vi "SMR_LabVIEW_V8.4.vi"() -> ()   [LabVIEW 2025]
uses:
  <vilib>/DAQmx/write.llb/DAQmx Write (Analog DBL 1Chan 1Samp).vi
  <vilib>/DAQmx/read.llb/DAQmx Read (Analog 1D DBL NChan 1Samp).vi
  <vilib>/DAQmx/read.llb/DAQmx Read (Analog 2D DBL NChan NSamp).vi
  <vilib>/Analysis/baseanly.llb/Mean (DBL).vi
  <vilib>/DAQmx/create/channels.llb/DAQmx Create Channel (AI-Temperature-Thermocouple).vi
  <vilib>/DAQmx/create/channels.llb/DAQmx Create Channel (AI-Voltage-Basic).vi
  <vilib>/DAQmx/create/channels.llb/DAQmx Create Channel (AO-Voltage-Basic).vi
  <vilib>/DAQmx/miscellaneous.llb/DAQmx Fill In Error Info.vi
  <vilib>/DAQmx/configure/timing.llb/DAQmx Timing (Sample Clock).vi
  <vilib>/addons/control/pid/pid.llb/PID (DBL).vi
  <vilib>/measure/maspectr.llb/FFT Power Spectrum and PSD for 1 Chan.vi
  <vilib>/measure/matone.llb/Extract Single Tone Information 1 Chan.vi
  <vilib>/addons/control/pid/NI_PID_pid.lvlib
  <vilib>/Analysis/NI_AALBase.lvlib
  <vilib>/ptbypt/NI_PtbyPt.lvlib
  <vilib>/measure/NI_MAPro.lvlib
panel:
  out "HW Valve Command (V)":dbl
  in  "HX Flow Setpoint (GPM)":dbl
  in  "Manual HW Valve Voltage (V)":dbl
  in  "HW Valve: Manual / PID":bool
  in  "PID gains for HW Valve":T1={"proportional gain (Kc)"=1.0, "integral time (Ti, min)"=0.01, "derivative time (Td, min)"=0.0} {"derivative time (Td, min)" format="%.3f"; "integral time (Ti, min)" format="%.3f"; "proportional gain (Kc)" format="%.3f"}
  out "Rod Power (W)":dbl
  out "Current Through Rod (A)":dbl
  out "Time in Steady State (s)":dbl
  in  "Steady-State Dwell (s)":dbl
  out "Main Loop Flow (GPM)":dbl
  out "FM Amplitude":dbl
  out "FM Frequency":dbl
  out "Spectrum":cluster{"f0":dbl, "df":dbl, "magnitude":dbl[]}(graph)
  out "Raw Signal":waveform(dbl)(graph)
  out "Smoothed HX Flow (GPM)":dbl
  out "Flow History":dbl(graph)
  out "HX Flow (GPM)":dbl
  out "Voltage Across Rod (V)":dbl format="%0.2f"
  out "Current Run Folder":path
  in  "Log Root Folder":path=path "C:/Users/LocalUser/Documents/GitHub/thermal-loop/resources/v0.1.1/data/001"
  out "Raw NI9201 \nVoltage Display":T2
  in  "Loop Period (ms)":dbl=1000.0
  in  "Stop":bool
  out "Auto Steady State Threshold (deg C/min)":dbl
  out "Max dT/dt (deg C/min)":dbl
  out "Temp Change Rate (deg C/min)":dbl
  out "5-Min Baseline Complete":bool
  out "Rate Window Ready":bool
  out "Steady State":bool
  in  "Voltage Limit (V)":dbl=10.0
  in  "Temperature Limit (C)":dbl=50.0
  in  "Pressure Limit (psi)":dbl=15.0
  out "Max Voltage":bool
  out "Max Temperature":bool
  out "Max Pressure":bool
  out "Heat Exchanger Pressure History":dbl(graph)
  out "Main Loop Pressure History":T3(graph)
  out "Overall Avg Pressure (psi)":dbl
  out "Heat Exchanger Pressure P6 (psi)":dbl
  out "Main Loop Avg Pressure (psi)":dbl
  out "Pressure Display":T4
  out "Overall Pressure History":T5(graph)
  out "Max Loop Pressure (psi)":dbl
  out "Heat Exchanger Temperature History":cluster{"Waveform":dbl, "Waveform":dbl}(graph)
  out "Main Loop Temeperature History":T6(graph)
  out "Heat Exchanger Avg Temp (deg C)":dbl
  out "Temperature Display":T7
  out "Overall Temperature History":T8(graph)
  out "Overall Avg Temp (deg C)":dbl
  out "Max Loop Temp (deg C)":dbl
  out "Final P-Valve Voltage (V)":dbl
  out "PID Trim Voltage (V)":dbl
  in  "PID Temp Setpoint (deg C)":dbl
  in  "Auto PID Enable":bool
  in  "Manual P-Valve Voltage (V)":dbl min=0.0 max=10.0
  out "Main Loop Avg Temp (deg C)":dbl
  # "HoneyWell Valve Control"
  # "Heat Exchanger Flow"
  # "Control/Troubleshoot"
  # "Steady State"
  # "Emergency Indicators"
  # "Pressure"
  # "Temperature"
  # "Proportional Valve Control"
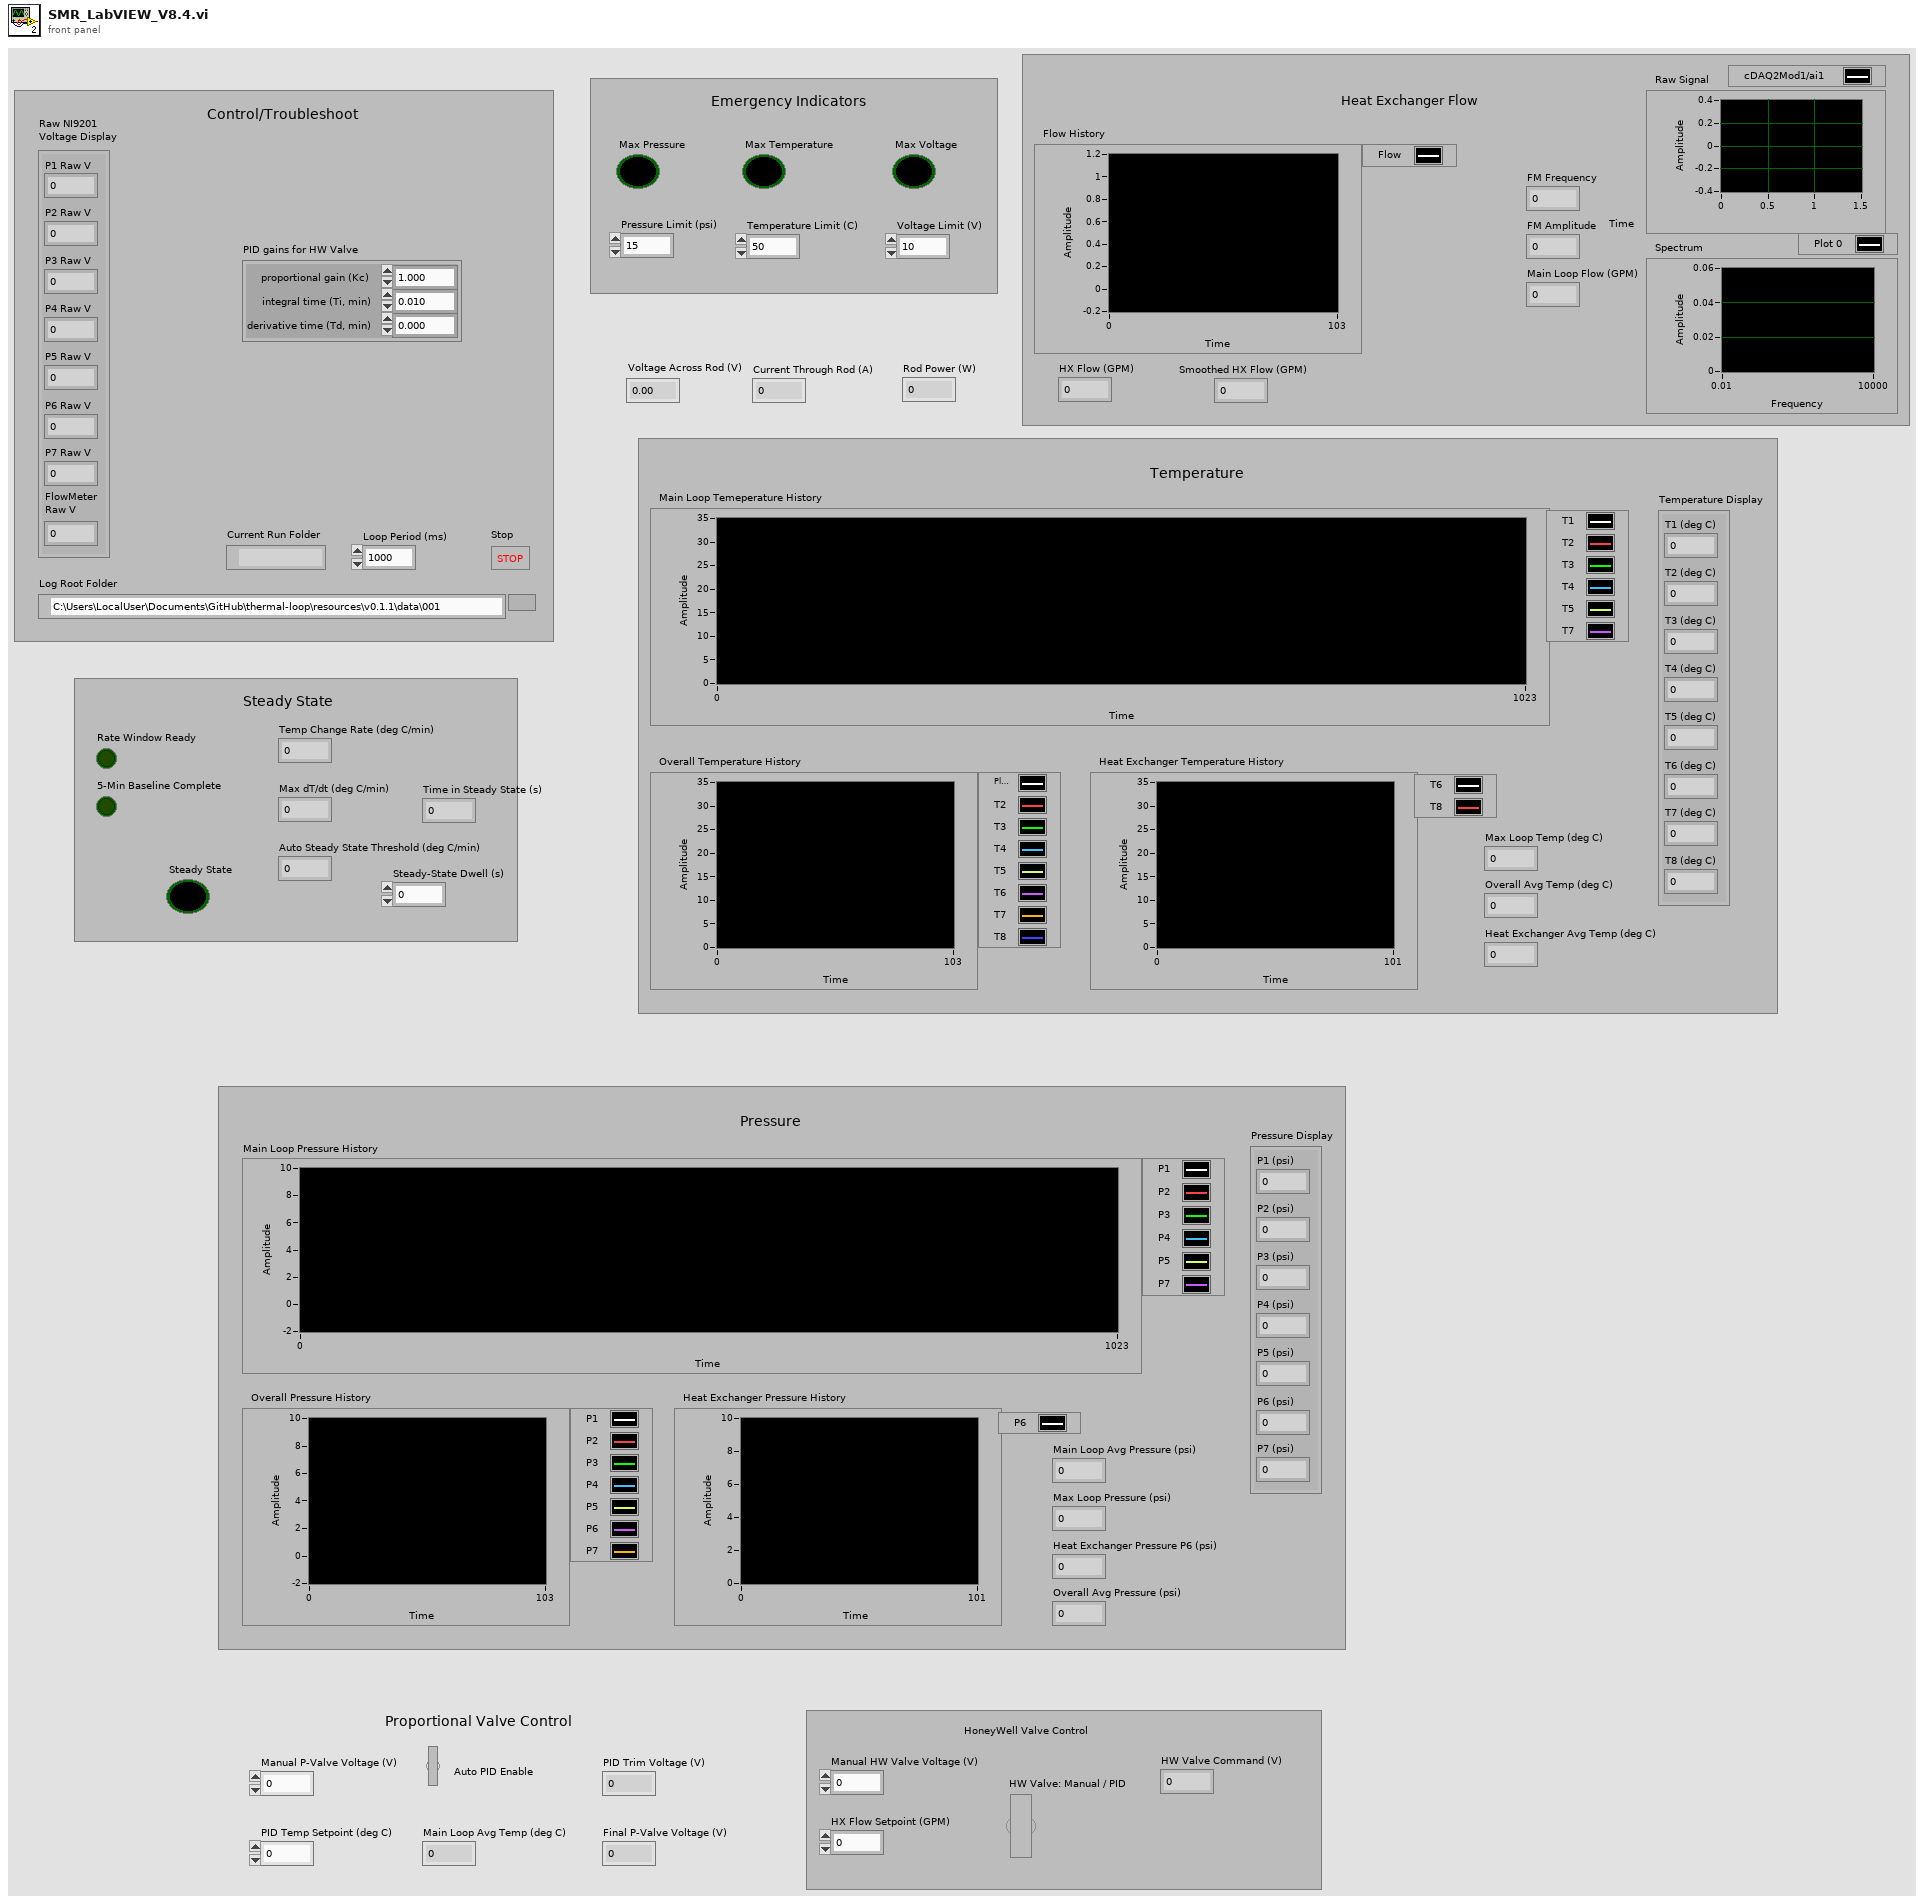
[diagram p1: front panel]
types:
  T1 = cluster{"proportional gain (Kc)":dbl, "integral time (Ti, min)":dbl, "derivative time (Td, min)":dbl}
  T2 = cluster{"P1 Raw V":dbl, "P2 Raw V":dbl, "P3 Raw V":dbl, "P4 Raw V":dbl, "P5 Raw V":dbl, "P6 Raw V":dbl, "P7 Raw V":dbl, "FlowMeter\nRaw V":dbl}
  T3 = cluster{"P1":dbl, "P2":dbl, "P3":dbl, "P4":dbl, "P5":dbl, "P7":dbl}
  T4 = cluster{"P1 (psi)":dbl, "P2 (psi)":dbl, "P3 (psi)":dbl, "P4 (psi)":dbl, "P5 (psi)":dbl, "P6 (psi)":dbl, "P7 (psi)":dbl}
  T5 = cluster{"P1":dbl, "P2":dbl, "P3":dbl, "P4":dbl, "P5":dbl, "P6":dbl, "P7":dbl}
  T6 = cluster{"Waveform":dbl, "Waveform":dbl, "Waveform":dbl, "Waveform":dbl, "Waveform":dbl, "Waveform":dbl}
  T7 = cluster{"T1 (deg C)":dbl, "T2 (deg C)":dbl, "T3 (deg C)":dbl, "T4 (deg C)":dbl, "T5 (deg C)":dbl, "T6 (deg C)":dbl, "T7 (deg C)":dbl, "T8 (deg C)":dbl}
  T8 = cluster{"Waveform":dbl, "Waveform":dbl, "Waveform":dbl, "Waveform":dbl, "Waveform":dbl, "Waveform":dbl, "Waveform":dbl, "Waveform":dbl}
  T9 = enum16{"open", "replace", "create", "open or create", "replace or create", "replace or create with confirmation"}
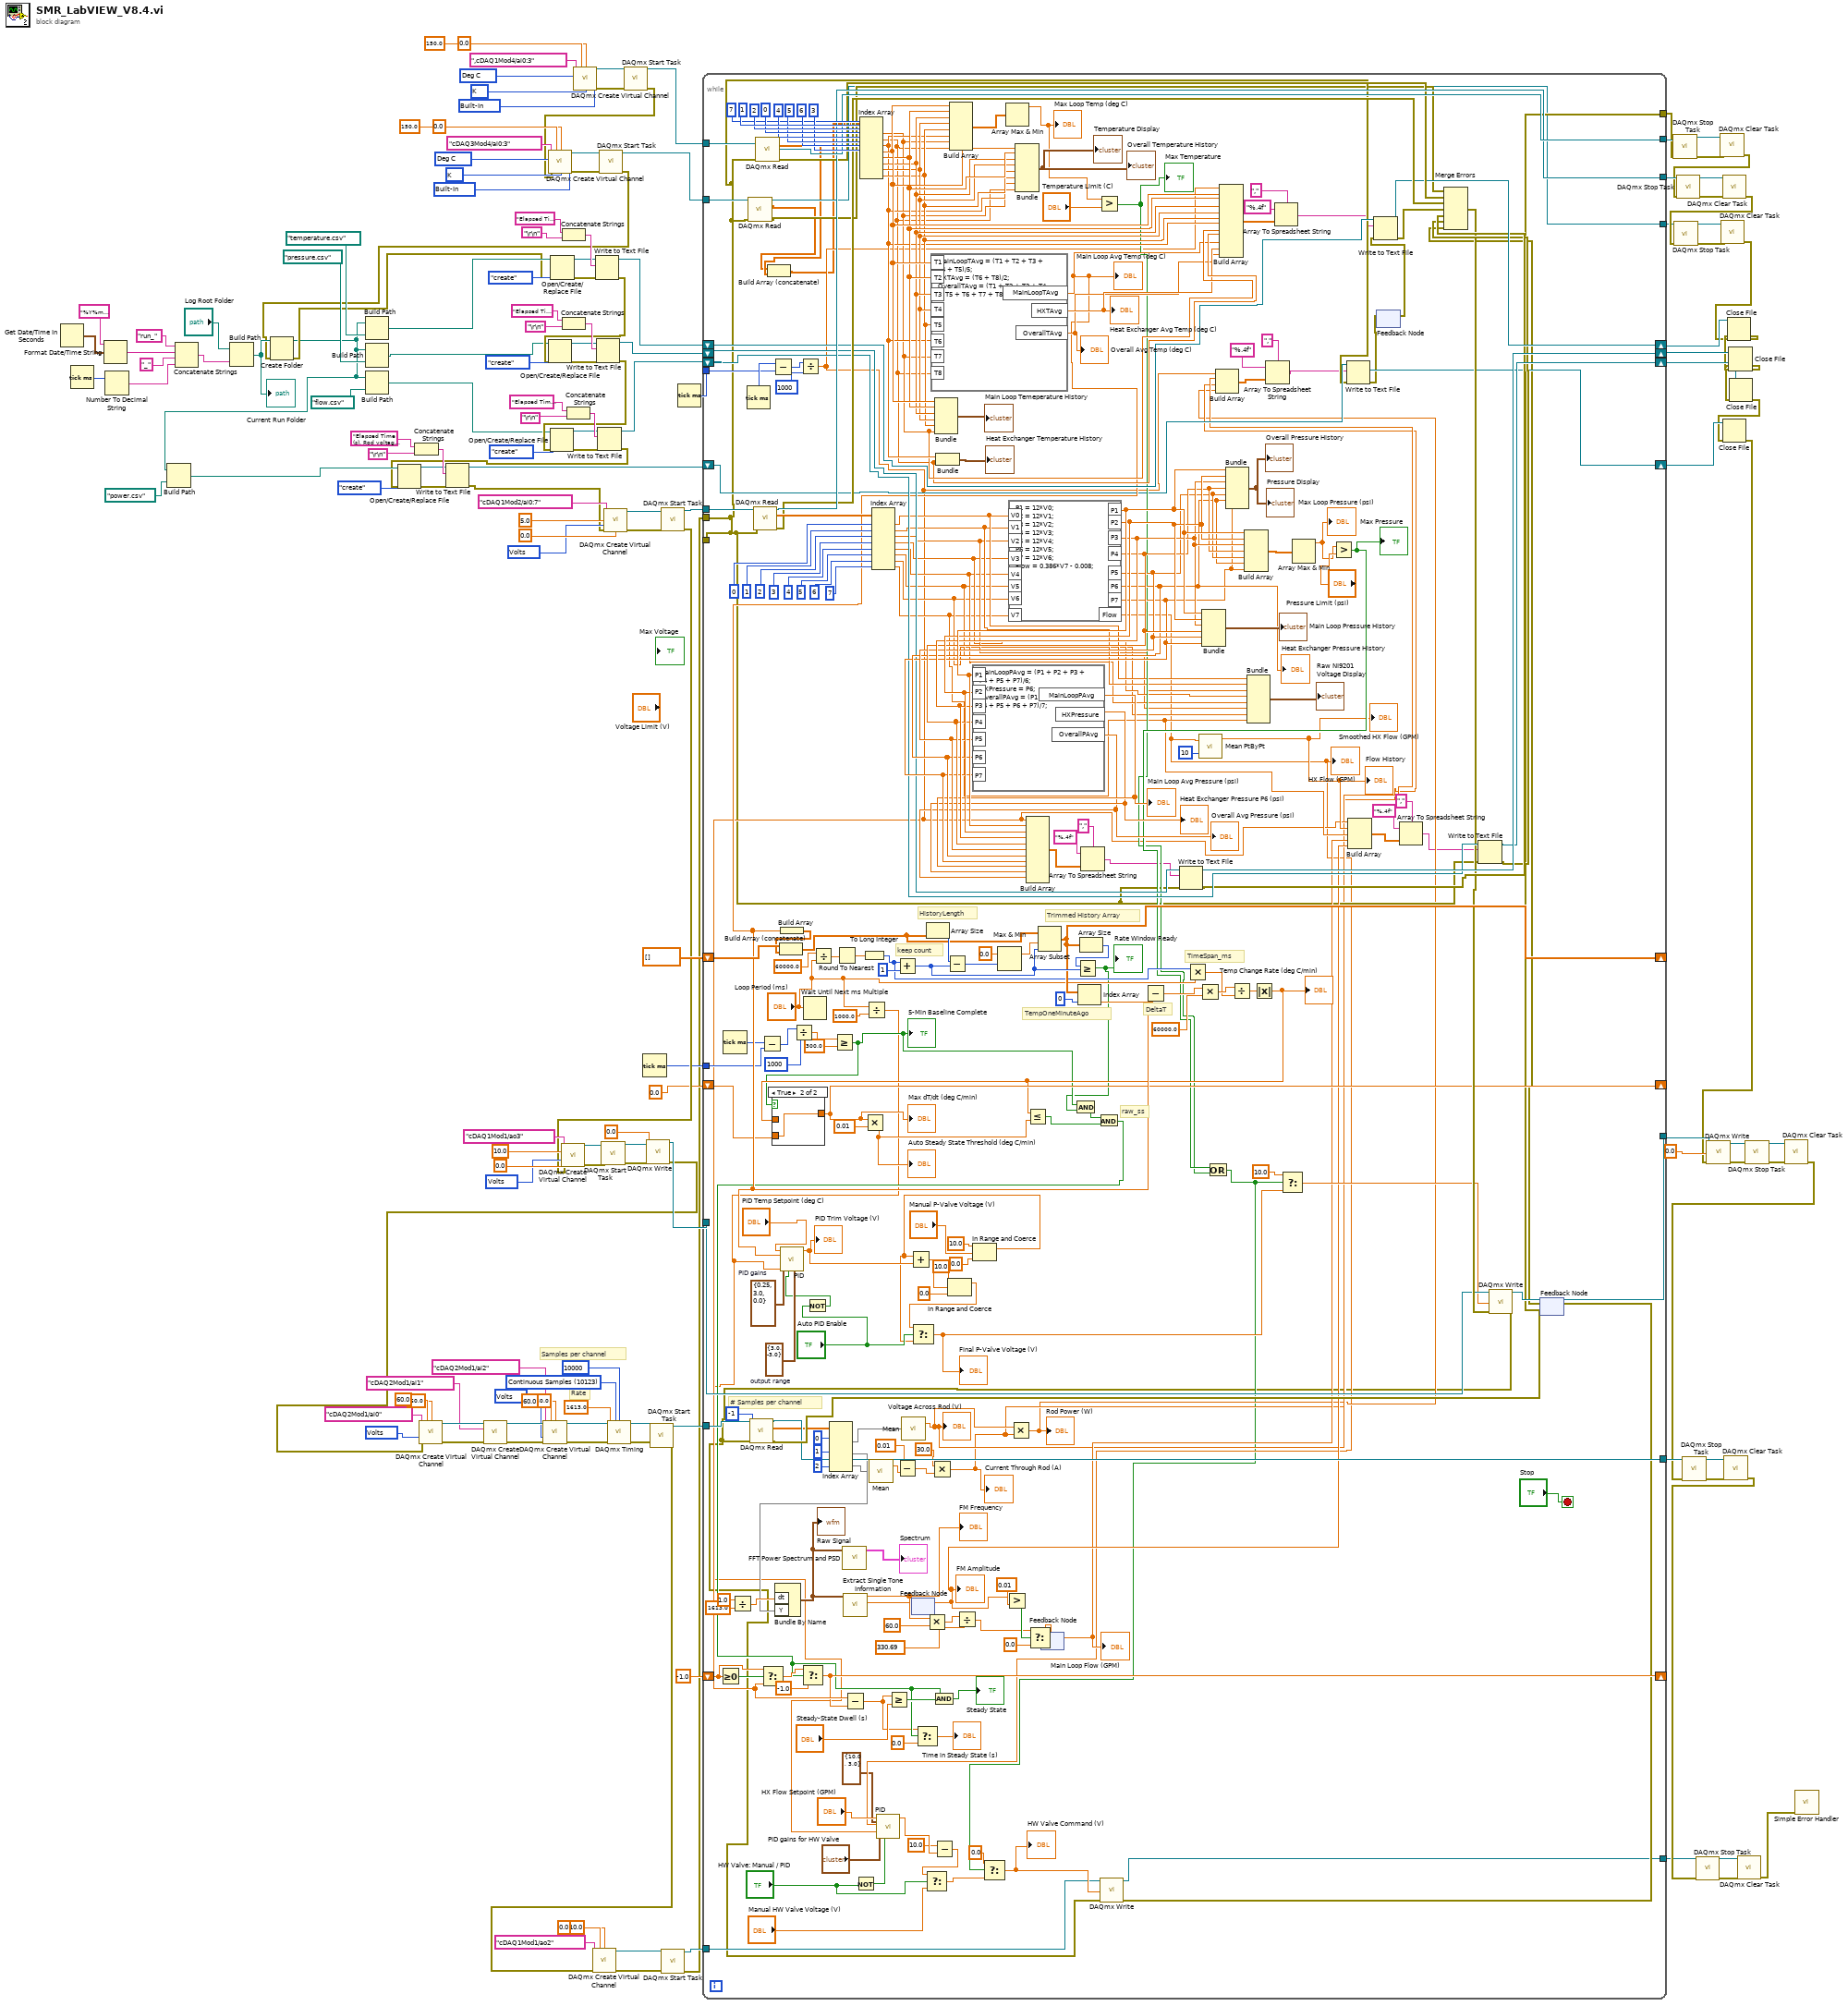
[diagram p0: block diagram]
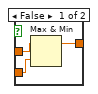
[diagram p2: hidden frame]
diagram:
  w17 = 10348 items=["Volts"=10348, "From Custom Scale"=10065] ("units")
  w34 = 10200 items=["Built-In"=10200, "Constant Value"=10116, "Channel"=10113] ("cjc source")
  w35 = 10073 items=["J"=10072, "K"=10073, "N"=10077, "R"=10082, "S"=10085, "T"=10086, "B"=10047, "E"=10055] ("thermocouple type")
  w36 = 10143 items=["Deg C"=10143, "Deg F"=10144, "Kelvins"=10325, "Deg R"=10145, "From Custom Scale"=10065] ("units")
  w66 = 10123 items=["Finite Samples"=10178, "Continuous Samples"=10123, "Hardware Timed Single Point"=12522] ("sample mode")
  w68 = 10348 items=["Volts"=10348, "From Custom Scale"=10065] ("units")
  w87 = 10348 items=["Volts"=10348, "From Custom Scale"=10065] ("units")
  w149 = 10200 items=["Built-In"=10200, "Constant Value"=10116, "Channel"=10113] ("cjc source")
  w150 = 10073 items=["J"=10072, "K"=10073, "N"=10077, "R"=10082, "S"=10085, "T"=10086, "B"=10047, "E"=10055] ("thermocouple type")
  w151 = 10143 items=["Deg C"=10143, "Deg F"=10144, "Kelvins"=10325, "Deg R"=10145, "From Custom Scale"=10065] ("units")
  w158 = 10348 items=["Volts"=10348, "From Custom Scale"=10065] ("units")
  # "Samples per channel"
  # "Rate"
  n1 = Get Date/Time In Seconds() -> (seconds since 1Jan1904=w108:timestamp)
  n2 = Tick Count (ms)() -> (millisecond timer value=w106:u32)
  n3 = Format Date/Time String(time format string (%c)="%Y%m%d_%H%M%S", seconds (now)=w108) -> (date/time string=w103:string)  [unwired: 1 in]
  n4 = Number To Decimal String(number=w106) -> (decimal integer string=w104:string)  [unwired: 1 in]
  n5 = Concatenate Strings("run_" ("string"), w103, "_" ("string"), w104) -> (w100:string)
  n6 = Build Path(base path="Log Root Folder", name or relative path=w100) -> (appended path=w99:path)
  "Current Run Folder" <- w99
  n7 = Concatenate Strings("Elapsed Time (s), Rod voltage (V), Rod Current (A), Rod Power (W)", "\r\n") -> (w53:string)
  n8 = Concatenate Strings("Elapsed Time (s),T1 (deg C),T2 (deg C),T3 (deg C),T4 (deg C),T5 (deg C),T6 (deg C),T7 (deg C),T8 (deg C),Main Loop Avg Temp (deg C),HX Avg Temp (deg C),Overall Avg Temp (deg C)", "\r\n") -> (w132:string)
  n9 = Concatenate Strings("Elapsed Time (s),P1 (psi),P2 (psi),P3 (psi),P4 (psi),P5 (psi),P6 (psi),P7 (psi),Main Loop Avg Pressure (psi),HX Pressure (psi),Overall Avg Pressure (psi)", "\r\n") -> (w130:string)
  n10 = Concatenate Strings("Elapsed Time (s),Heat Exchanger Flow (GPM),Flow Raw Voltage (V), Main Loop Flow (GPM), Flow Signal Amplitude (V)", "\r\n") -> (w126:string)
  n11 = call-poly <vilib>:"DAQmx Create Virtual Channel.vi"("maximum value"=150.0, "minimum value"=0.0, "physical channels"=tag ",cDAQ1Mod4/ai0:3", "cjc source"=w149, "units"=w151, "thermocouple type"=w150) -> ("task out"=w148:refnum<k21>, "error out"=w147:errorcluster)  [unwired: 8 in]
  n12 = call <vilib>:"DAQmx Start Task.vi"("task/channels in"=w148, "error in"=w147) -> ("task out"=w146:refnum<k21>, "error out"=w30:errorcluster)  [unwired: 12 in]
  n13 = call-poly <vilib>:"DAQmx Create Virtual Channel.vi"("maximum value"=150.0, "minimum value"=0.0, "physical channels"=tag "cDAQ3Mod4/ai0:3", "cjc source"=w34, "units"=w36, "error in"=w30, "thermocouple type"=w35) -> ("task out"=w33:refnum<k21>, "error out"=w32:errorcluster)  [unwired: 7 in]
  n14 = call <vilib>:"DAQmx Start Task.vi"("task/channels in"=w33, "error in"=w32) -> ("task out"=w28:refnum<k21>, "error out"=w29:errorcluster)  [unwired: 12 in]
  n15 = Create Folder(path (use dialog)=w99, error in=w29) -> (created path=w47:path, error out=w92:errorcluster)  [unwired: 1 in, 1 out]
  n16 = Build Path(base path=w47, name or relative path=path "power.csv") -> (appended path=w48:path)
  n17 = Build Path(base path=w47, name or relative path=path "temperature.csv") -> (appended path=w98:path)
  n18 = Build Path(base path=w47, name or relative path=path "pressure.csv") -> (appended path=w97:path)
  n19 = Build Path(base path=w47, name or relative path=path "flow.csv") -> (appended path=w96:path)
  n20 = Open/Create/Replace File(file path (use dialog)=w98, error in=w92, operation (0:open)=T9."create") -> (refnum out=w131:refnum<file>, error out=w115:errorcluster)  [unwired: 3 in, 1 out]
  n21 = Write to Text File(file (use dialog)=w131, text=w132, error in=w115) -> (refnum out=w122:refnum<file>, error out=w114:errorcluster)  [unwired: 1 in, 1 out]
  n22 = Open/Create/Replace File(file path (use dialog)=w97, error in=w114, operation (0:open)=T9."create") -> (refnum out=w129:refnum<file>, error out=w113:errorcluster)  [unwired: 3 in, 1 out]
  n23 = Write to Text File(file (use dialog)=w129, text=w130, error in=w113) -> (refnum out=w121:refnum<file>, error out=w112:errorcluster)  [unwired: 1 in, 1 out]
  n24 = Open/Create/Replace File(file path (use dialog)=w96, error in=w112, operation (0:open)=T9."create") -> (refnum out=w125:refnum<file>, error out=w111:errorcluster)  [unwired: 3 in, 1 out]
  n25 = Write to Text File(file (use dialog)=w125, text=w126, error in=w111) -> (refnum out=w120:refnum<file>, error out=w45:errorcluster)  [unwired: 1 in, 1 out]
  n26 = Open/Create/Replace File(file path (use dialog)=w48, error in=w45, operation (0:open)=T9."create") -> (refnum out=w52:refnum<file>, error out=w49:errorcluster)  [unwired: 3 in, 1 out]
  n27 = Write to Text File(file (use dialog)=w52, text=w53, error in=w49) -> (refnum out=w43:refnum<file>, error out=w44:errorcluster)  [unwired: 1 in, 1 out]
  n28 = call-poly <vilib>:"DAQmx Create Virtual Channel.vi"("maximum value"=5.0, "minimum value"=0.0, "physical channels"=tag "cDAQ1Mod2/ai0:7", "units"=w158, "error in"=w44) -> ("task out"=w157:refnum<k21>, "error out"=w156:errorcluster)  [unwired: 9 in]
  n29 = Tick Count (ms)() -> (millisecond timer value=w73:u32)
  n30 = call <vilib>:"DAQmx Start Task.vi"("task/channels in"=w157, "error in"=w156) -> ("task out"=w155:refnum<k21>, "error out"=w80:errorcluster)  [unwired: 12 in]
  n31 = call-poly <vilib>:"DAQmx Create Virtual Channel.vi"("maximum value"=10.0, "minimum value"=0.0, "physical channels"=tag "cDAQ1Mod1/ao3", "units"=w87, "error in"=w80) -> ("task out"=w86:refnum<k21>, "error out"=w85:errorcluster)  [unwired: 9 in]
  n32 = call <vilib>:"DAQmx Start Task.vi"("task/channels in"=w86, "error in"=w85) -> ("task out"=w84:refnum<k21>, "error out"=w83:errorcluster)  [unwired: 12 in]
  n33 = call-poly <vilib>:"DAQmx Write.vi"("task/channels in"=w84, "data"=0.0, "error in"=w83) -> ("task out"=w81:refnum<k21>, "error out"=w60:errorcluster)  [unwired: 10 in, 1 out]
  n34 = call-poly <vilib>:"DAQmx Create Virtual Channel.vi"("maximum value"=60.0, "minimum value"=-60.0, "physical channels"=tag "cDAQ2Mod1/ai0", "units"=w68, "error in"=w60) -> ("task out"=w57:refnum<k21>, "error out"=w56:errorcluster)  [unwired: 9 in]
  n35 = call-poly <vilib>:"DAQmx Create Virtual Channel.vi"("task in"=w57, "physical channels"=tag "cDAQ2Mod1/ai1", "error in"=w56) -> ("task out"=w21:refnum<k21>, "error out"=w19:errorcluster)  [unwired: 11 in]
  n36 = call-poly <vilib>:"DAQmx Create Virtual Channel.vi"("task in"=w21, "maximum value"=60.0, "minimum value"=-60.0, "physical channels"=tag "cDAQ2Mod1/ai2", "units"=w17, "error in"=w19) -> ("task out"=w20:refnum<k21>, "error out"=w18:errorcluster)  [unwired: 8 in]
  n37 = call-poly <vilib>:"DAQmx Timing.vi"("task/channels in"=w20, "sample mode"=w66, "samples per channel"=10000, "rate"=1613.0, "error in"=w18) -> ("task out"=w64:refnum<k21>, "error out"=w63:errorcluster)  [unwired: 9 in]
  n38 = call <vilib>:"DAQmx Start Task.vi"("task/channels in"=w64, "error in"=w63) -> ("task out"=w59:refnum<k21>, "error out"=w8:errorcluster)  [unwired: 12 in]
  n39 = call-poly <vilib>:"DAQmx Create Virtual Channel.vi"("maximum value"=10.0, "minimum value"=0.0, "physical channels"=tag "cDAQ1Mod1/ao2", "error in"=w8) -> ("task out"=w11:refnum<k21>, "error out"=w10:errorcluster)  [unwired: 10 in]
  n40 = call <vilib>:"DAQmx Start Task.vi"("task/channels in"=w11, "error in"=w10) -> ("task out"=w9:refnum<k21>, "error out"=w7:errorcluster)  [unwired: 12 in]
  n41 = Tick Count (ms)() -> (millisecond timer value=w119:u32)
  n42 = while {
    tunnel: w155 -> [w395]
    tunnel: w146 -> [w378]
    tunnel: [w369] -> w145
    tunnel: [w200] -> _
    tunnel: [w368] -> w144
    tunnel: [w256] -> w143
    shift-right: [w347] -> w118
    shift-left: w122 -> [w348]
    shift-right: [w332] -> w117
    shift-left: w121 -> [w333]
    shift-right: [w327] -> w116
    shift-left: w120 -> [w328]
    tunnel: w119 -> [w364]
    shift-right: [w306] -> _
    shift-left: dbl[] [] -> [w319]
    tunnel: w81 -> [w288]
    tunnel: w7 -> [w200]
    tunnel: [w294] -> w78
    tunnel: w73 -> [w277]
    shift-right: [w270] -> _
    shift-left: 0.0 -> [w272]
    tunnel: w59 -> [w255]
    tunnel: [w254] -> w58
    shift-right: [w217] -> w42
    shift-left: w43 -> [w218]
    shift-right: [w209] -> _
    shift-left: -1.0 -> [w213]
    tunnel: w28 -> [w201]
    tunnel: [w198] -> w24
    tunnel: w9 -> [w171]
    tunnel: [w167] -> w2
    stop <- "Stop" stop-if-true
    w292 = cluster{"output high":dbl, "output low":dbl} {"output high"=3.0, "output low"=-3.0}  # output range
    w293 = T1 {"proportional gain (Kc)"=0.25, "integral time (Ti, min)"=3.0, "derivative time (Td, min)"=0.0}  # PID gains
    # "raw_ss"
    # "# Samples per channel"
    # "TimeSpan_ms"
    # "DeltaT"
    # "TempOneMinuteAgo"
    # "Trimmed History Array"
    # "HistoryLength"
    # "keep count"
    n43 = Greater Or Equal To 0?(x=w213) -> (x >= 0?=w214:bool)
    n44 = Tick Count (ms)() -> (millisecond timer value=w278:u32)
    n45 = Divide(x=1.0, y=1613.0) -> (x/y=w228:dbl)
    n46 = Tick Count (ms)() -> (millisecond timer value=w365:u32)
    n47 = call-poly <vilib>:"DAQmx Read.vi"("task/channels in"=w201, "error in"=w200) -> ("task out"=w198:refnum<k21>, "data"=w195:dbl[], "error out"=w199:errorcluster)  [unwired: 11 in]
    n48 = call-poly <vilib>:"DAQmx Read.vi"("task/channels in"=w395, "error in"=w200) -> ("task out"=w368:refnum<k21>, "data"=w386:dbl[], "error out"=w366:errorcluster)  [unwired: 11 in]
    n49 = call-poly <vilib>:"DAQmx Read.vi"("task/channels in"=w378, "error in"=w200) -> ("task out"=w369:refnum<k21>, "data"=w196:dbl[], "error out"=w367:errorcluster)  [unwired: 11 in]
    n50 = Subtract(x=w278, y=w277) -> (x-y=w276:u32)
    n51 = Build Array (concatenate)(w195, w196) -> (w197:dbl[])
    n52 = Subtract(x=w365, y=w364) -> (x-y=w363:u32)
    n53 = Divide(x=w276, y=u32 1000) -> (x/y=w274:dbl)
    n54 = Divide(x=w363, y=u32 1000) -> (x/y=w210:dbl)
    n55 = Select(t=w213, s=w214, f=w210) -> (s? t:f=w212:dbl)
    n56 = Wait Until Next ms Multiple(millisecond multiple="Loop Period (ms)") -> ()  [unwired: 1 out]
    n57 = Not(x="Auto PID Enable") -> (.not. x?=w289:bool)
    n58 = Divide(x=60000.0, y="Loop Period (ms)") -> (x/y=w316:dbl)
    n59 = Greater Or Equal?(x=w274, y=300.0) -> (x >= y?=w267:bool)
    "5-Min Baseline Complete" <- w267
    n60 = Round To Nearest(number=w316) -> (nearest integer value=w315:dbl)
    n61 = Not(x="HW Valve: Manual / PID") -> (.not. x?=w181:bool)
    n62 = Index Array(array=w197, index #1=7 ("index"), index #2=1 ("index"), index #3=2 ("index"), index #4=0 ("index"), index #5=4 ("index"), index #6=5 ("index"), index #7=6 ("index"), index #8=3 ("index")) -> (element #1=w355:dbl, element #2=w354:dbl, element #3=w356:dbl, element #4=w361:dbl, element #5=w360:dbl, element #6=w359:dbl, element #7=w358:dbl, element #8=w357:dbl)
    n63 = To Long Integer(number=w315) -> (32bit integer=w303:i32)
    n64 = Divide(x="Loop Period (ms)", y=1000.0) -> (x/y=w166:dbl)
    n65 = Index Array(array=w386, index #1=0 ("index"), index #2=1 ("index"), index #3=2 ("index"), index #4=3 ("index"), index #5=4 ("index"), index #6=5 ("index"), index #7=6 ("index"), index #8=7 ("index")) -> (element #1=w253:dbl, element #2=w252:dbl, element #3=w251:dbl, element #4=w250:dbl, element #5=w249:dbl, element #6=w248:dbl, element #7=w247:dbl, element #8=w246:dbl)
    n66 = Add(x=w303, y=1) -> (x+y=w308:i32)
    n67 = feedback #1() -> (w224:dbl)  [unwired: 1 in]
    "FM Amplitude" <- w224
    n68 = formula code="MainLoopTAvg = (T1 + T2 + T3 + T4 + T5)/5;\nHXTAvg = (T6 + T8)/2;\nOverallTAvg = (T1 + T2 + T3 + T4 + T5 + T6 + T7 + T8)/8;"("T1"=w361, "T2"=w360, "T3"=w359, "T4"=w358, "T5"=w357, "T6"=w356, "T7"=w355, "T8"=w354) -> ("MainLoopTAvg"=w280:dbl, "HXTAvg"=w353:dbl, "OverallTAvg"=w352:dbl)
    "Overall Avg Temp (deg C)" <- w352
    "Main Loop Avg Temp (deg C)" <- w280
    "Heat Exchanger Avg Temp (deg C)" <- w353
    n69 = Build Array(w280) -> (w318:dbl[])
    n70 = Build Array (concatenate)(w319, w318) -> (w310:dbl[])
    n71 = call-poly <vilib>:"PID.vi"("reinitialize? (F)"=w289, "output range"=w292, "dt (s)"=w166, "PID gains"=w293, "process variable"=w280, "setpoint"="PID Temp Setpoint (deg C)") -> ("output"=w287:dbl)  [unwired: 4 in, 1 out]
    "PID Trim Voltage (V)" <- w287
    n72 = Array Size(array=w310) -> (size(s)=w313:i32)
    n73 = Bundle("Waveform"=w361, "Waveform"=w360, "Waveform"=w359, "Waveform"=w358, "Waveform"=w357, "Waveform"=w355) -> (→"Main Loop Temeperature History":T6)  [unwired: 1 in]
    n74 = Bundle("Waveform"=w356, "Waveform"=w354) -> (→"Heat Exchanger Temperature History":cluster{"Waveform":dbl, "Waveform":dbl})  [unwired: 1 in]
    n75 = Subtract(x=w313, y=w308) -> (x-y=w311:i32)
    n76 = Build Array(w361, w360, w359, w358, w357, w356, w355, w354) -> (w396:dbl[])
    n77 = In Range and Coerce(upper limit=10.0, x="Manual P-Valve Voltage (V)", lower limit=0.0) -> (coerced(x)=w282:dbl)  [unwired: 1 out]
    n78 = Add(x=w282, y=w287) -> (x+y=w286:dbl)
    n79 = In Range and Coerce(upper limit=10.0, x=w286, lower limit=0.0) -> (coerced(x)=w281:dbl)  [unwired: 1 out]
    n80 = Select(t=w281, s="Auto PID Enable", f=w282) -> (s? t:f=w259:dbl)
    "Final P-Valve Voltage (V)" <- w259
    n81 = Max & Min(x=0.0, y=w311) -> (max(x,y)=w309:dbl)  [unwired: 1 out]
    n82 = Array Max & Min(array=w396) -> (max value=w321:dbl)  [unwired: 3 out]
    "Max Loop Temp (deg C)" <- w321
    n83 = Greater?(x=w224, y=0.01) -> (0:w232:bool)
    n84 = formula code="P1 = 12*V0;\nP2 = 12*V1;\nP3 = 12*V2;\nP4 = 12*V3;\nP5 = 12*V4;\nP6 = 12*V5; \nP7 = 12*V6;\nFlow = 0.386*V7 - 0.008;"("V0"=w253, "V1"=w252, "V2"=w251, "V3"=w250, "V4"=w249, "V5"=w248, "V6"=w247, "V7"=w246) -> ("P1"=w346:dbl, "P2"=w345:dbl, "P3"=w344:dbl, "P4"=w343:dbl, "P5"=w342:dbl, "P6"=w341:dbl, "P7"=w340:dbl, "Flow"=w184:dbl)
    "HX Flow (GPM)" <- w184
    "Heat Exchanger Pressure History" <- w341
    n85 = call-poly <vilib>:"PID.vi"("reinitialize? (F)"=w181, "output range"=cluster{"output high":dbl, "output low":dbl} {"output high"=10.0, "output low"=3.0}, "dt (s)"=w166, "PID gains"="PID gains for HW Valve", "process variable"=w184, "setpoint"="HX Flow Setpoint (GPM)") -> ("output"=w180:dbl)  [unwired: 4 in, 1 out]
    n86 = Subtract(x=10.0, y=w180) -> (x-y=w177:dbl)
    n87 = Select(t=w177, s="HW Valve: Manual / PID", f="Manual HW Valve Voltage (V)") -> (s? t:f=w174:dbl)
    n88 = formula code="MainLoopPAvg = (P1 + P2 + P3 + P4 + P5 + P7)/6;\nHXPressure = P6;\nOverallPAvg = (P1 + P2 + P3 + P4 + P5 + P6 + P7)/7;"("P1"=w346, "P2"=w345, "P3"=w344, "P4"=w343, "P5"=w342, "P6"=w341, "P7"=w340) -> ("MainLoopPAvg"=w339:dbl, "HXPressure"=w338:dbl, "OverallPAvg"=w337:dbl)
    "Overall Avg Pressure (psi)" <- w337
    "Heat Exchanger Pressure P6 (psi)" <- w338
    "Main Loop Avg Pressure (psi)" <- w339
    n89 = Bundle("Waveform"=w361, "Waveform"=w360, "Waveform"=w359, "Waveform"=w358, "Waveform"=w357, "Waveform"=w356, "Waveform"=w355, "Waveform"=w354) -> (→"Overall Temperature History" →"Temperature Display":T8)  [unwired: 1 in]
    n90 = Build Array(w210, w346, w345, w344, w343, w342, w341, w340, w339, w338, w337) -> (w336:dbl[])
    n91 = Array Subset(array=w310, index=w309, length=w308) -> (w306:dbl[])
    n92 = feedback #2() -> (w222:dbl)  [unwired: 1 in]
    "Main Loop Flow (GPM)" <- w222
    n93 = Index Array(array=w306, index=0) -> (element=w304:dbl)
    n94 = Array Size(array=w306) -> (size(s)=w307:i32)
    n95 = Greater Or Equal?(x=w307, y=w308) -> (x >= y?=w266:bool)
    "Rate Window Ready" <- w266
    n96 = And(x=w267, y=w266) -> (x .and. y?=w265:bool)
    n97 = Array To Spreadsheet String(delimiter (Tab)=",", array=w336, 3:"%.4f" ("format string")) -> (spreadsheet string=w162:string)
    n98 = Greater?(x=w321, y="Temperature Limit (C)") -> (0:w262:bool)
    "Max Temperature" <- w262
    n99 = Subtract(x=w280, y=w304) -> (x-y=w302:dbl)
    n100 = Write to Text File(file (use dialog)=w333, text=w162, error in=w200) -> (refnum out=w332:refnum<file>, error out=w325:errorcluster)  [unwired: 1 in, 1 out]
    n101 = Multiply(x=w303, y="Loop Period (ms)") -> (x*y=w299:dbl)
    n102 = Multiply(x=w302, y=60000.0) -> (x*y=w300:dbl)
    n103 = call <vilib>:"Mean PtByPt.vi"("x"=w184, "sample length"=10) -> ("mean"=w244:dbl)  [unwired: 2 in, 1 out]
    "Flow History" <- w244
    "Smoothed HX Flow (GPM)" <- w244
    n104 = Bundle("P1"=w346, "P2"=w345, "P3"=w344, "P4"=w343, "P5"=w342, "P7"=w340) -> (→"Main Loop Pressure History":T3)  [unwired: 1 in]
    n105 = Build Array(w210, w361, w360, w359, w358, w357, w356, w355, w354, w280, w353, w352) -> (w351:dbl[])
    n106 = Bundle("P1"=w346, "P2"=w345, "P3"=w344, "P4"=w343, "P5"=w342, "P6"=w341, "P7"=w340) -> (→"Overall Pressure History" →"Pressure Display":T5)  [unwired: 1 in]
    n107 = Divide(x=w300, y=w299) -> (x/y=w298:dbl)
    n108 = Build Array(w346, w345, w344, w343, w342, w341, w340) -> (w385:dbl[])
    n109 = Bundle("Waveform"=w253, "Waveform"=w252, "Waveform"=w251, "Waveform"=w250, "Waveform"=w249, "Waveform"=w248, "Waveform"=w247, "Waveform"=w246) -> (→"Raw NI9201 \nVoltage Display":T8)  [unwired: 1 in]
    n110 = Absolute Value(x=w298) -> (abs(x)=w269:dbl)
    "Temp Change Rate (deg C/min)" <- w269
    n111 = case shown="True" w267 {
      tunnel: w272 -> [w400 w401]
      tunnel: w269 -> [w399 _]
      tunnel: [w398 w401] -> w270
      frame False {
        n112 = Max & Min(x=w399, y=w400) -> (max(x,y)=w398:dbl)  [unwired: 1 out]
      }
      frame True {
      }
    }
    "Max dT/dt (deg C/min)" <- w270
    n113 = Multiply(x=w270, y=0.01) -> (x*y=w268:dbl)
    "Auto Steady State Threshold (deg C/min)" <- w268
    n114 = Less Or Equal?(x=w269, y=w268) -> (x <= y?=w264:bool)
    n115 = And(x=w265, y=w264) -> (x .and. y?=w205:bool)
    n116 = Select(t=w212, s=w205, f=-1.0) -> (s? t:f=w209:dbl)
    n117 = Subtract(x=w210, y=w209) -> (x-y=w204:dbl)
    n118 = Greater Or Equal?(x=w204, y="Steady-State Dwell (s)") -> (x >= y?=w207:bool)
    n119 = Select(t=w204, s=w205, f=0.0) -> (s? t:f=→"Time in Steady State (s)":dbl)
    n120 = And(x=w205, y=w207) -> (x .and. y?=→"Steady State":bool)
    n121 = Array To Spreadsheet String(delimiter (Tab)=",", array=w351, 3:"%.4f" ("format string")) -> (spreadsheet string=w163:string)
    n122 = Array Max & Min(array=w385) -> (max value=w322:dbl)  [unwired: 3 out]
    "Max Loop Pressure (psi)" <- w322
    n123 = Greater?(x=w322, y="Pressure Limit (psi)") -> (0:w263:bool)
    "Max Pressure" <- w263
    n124 = Or(x=w263, y=w262) -> (x .or. y?=w175:bool)
    n125 = Select(t=0.0, s=w175, f=w174) -> (s? t:f=w172:dbl)
    "HW Valve Command (V)" <- w172
    n126 = Select(t=10.0, s=w175, f=w259) -> (s? t:f=w258:dbl)
    n127 = Build Array(w210, w244, w246, w222, w224) -> (w331:dbl[])
    n128 = feedback #3() -> (w215:errorcluster)  [unwired: 1 in]
    n129 = Write to Text File(file (use dialog)=w348, text=w163, error in=w215) -> (refnum out=w347:refnum<file>, error out=w326:errorcluster)  [unwired: 1 in, 1 out]
    n130 = Array To Spreadsheet String(delimiter (Tab)=",", array=w331, 3:"%.4f" ("format string")) -> (spreadsheet string=w165:string)
    n131 = Write to Text File(file (use dialog)=w328, text=w165, error in=w200) -> (refnum out=w327:refnum<file>, error out=w324:errorcluster)  [unwired: 1 in, 1 out]
    n132 = feedback #4() -> (w168:errorcluster)  [unwired: 1 in]
    n133 = Merge Errors(w199, w367, w366, w326, w325, w324, w168) -> (w295:errorcluster)
    n134 = call-poly <vilib>:"DAQmx Write.vi"("task/channels in"=w288, "data"=w258, "error in"=w295) -> ("task out"=w294:refnum<k21>, "error out"=w170:errorcluster)  [unwired: 10 in, 1 out]
    n135 = call-poly <vilib>:"DAQmx Read.vi"("task/channels in"=w255, "number of samples per channel"=-1, "error in"=w170) -> ("task out"=w254:refnum<k21>, "data"=w243:dbl[][], "error out"=w256:errorcluster)  [unwired: 10 in]
    n136 = Index Array(array=w243, index (row) #1=0 ("index (row)"), index (row) #2=1 ("index (row)"), index (row) #3=2 ("index (row)")) -> (element #1=w242:dbl[], element #2=w227:dbl[], element #3=w190:dbl[])  [unwired: 3 in]
    n137 = Bundle By Name("dt"=w228, "Y"=w227) -> (w226:waveform(dbl))  [unwired: 1 in]
    "Raw Signal" <- w226
    n138 = call-poly <vilib>:"FFT Power Spectrum and PSD.vi"("time signal"=w226) -> ("Power Spectrum / PSD"=→"Spectrum":cluster{"f0":dbl, "df":dbl, "magnitude":dbl[]})  [unwired: 7 in, 3 out]
    n139 = call-poly <vilib>:"Extract Single Tone Information.vi"("time signal in"=w226) -> ("detected amplitude"=w225:dbl, "detected frequency"=w238:dbl)  [unwired: 5 in, 4 out]
    "FM Frequency" <- w238
    n140 = call-poly <vilib>:"Mean.vi"("X"=w190) -> ("mean"=w191:dbl)  [unwired: 1 out]
    n141 = Subtract(x=0.01, y=w191) -> (x-y=w192:dbl)
    n142 = call-poly <vilib>:"Mean.vi"("X"=w242) -> ("mean"=w188:dbl)  [unwired: 1 out]
    "Voltage Across Rod (V)" <- w188
    n143 = feedback-in #1(w225) -> ()
    n144 = Multiply(x=w238, y=60.0) -> (x*y=w236:dbl)
    n145 = Multiply(x=30.0, y=w192) -> (x*y=w187:dbl)
    "Current Through Rod (A)" <- w187
    n146 = Divide(x=w236, y=330.69) -> (x/y=w231:dbl)
    n147 = Multiply(x=w188, y=w187) -> (x*y=w186:dbl)
    "Rod Power (W)" <- w186
    n148 = Select(t=w231, s=w232, f=0.0) -> (s? t:f=w223:dbl)
    n149 = feedback-in #2(w223) -> ()
    n150 = call-poly <vilib>:"DAQmx Write.vi"("task/channels in"=w171, "data"=w172, "error in"=w170) -> ("task out"=w167:refnum<k21>, "error out"=w169:errorcluster)  [unwired: 10 in, 1 out]
    n151 = Build Array(w210, w188, w187, w186) -> (w219:dbl[])
    n152 = Array To Spreadsheet String(delimiter (Tab)=",", array=w219, 3:"%.4f" ("format string")) -> (spreadsheet string=w164:string)
    n153 = Write to Text File(file (use dialog)=w218, text=w164, error in=w200) -> (refnum out=w217:refnum<file>, error out=w216:errorcluster)  [unwired: 1 in, 1 out]
    n154 = feedback-in #3(w216) -> ()
    n155 = feedback-in #4(w169) -> ()
  }
  n156 = call <vilib>:"DAQmx Stop Task.vi"("task/channels in"=w145, "error in"=w143) -> ("task out"=w142:refnum<k21>, "error out"=w140:errorcluster)  [unwired: 12 in]
  n157 = call <vilib>:"DAQmx Clear Task.vi"("task in"=w142, "error in"=w140) -> ("error out"=w139:errorcluster)  [unwired: 13 in]
  n158 = call <vilib>:"DAQmx Stop Task.vi"("task/channels in"=w144, "error in"=w139) -> ("task out"=w141:refnum<k21>, "error out"=w138:errorcluster)  [unwired: 12 in]
  n159 = call <vilib>:"DAQmx Clear Task.vi"("task in"=w141, "error in"=w138) -> ("error out"=w27:errorcluster)  [unwired: 13 in]
  n160 = call <vilib>:"DAQmx Stop Task.vi"("task/channels in"=w24, "error in"=w27) -> ("task out"=w23:refnum<k21>, "error out"=w26:errorcluster)  [unwired: 12 in]
  n161 = call <vilib>:"DAQmx Clear Task.vi"("task in"=w23, "error in"=w26) -> ("error out"=w25:errorcluster)  [unwired: 13 in]
  n162 = Close File(refnum=w118, error in=w25) -> (error out=w110:errorcluster)  [unwired: 1 out]
  n163 = Close File(refnum=w117, error in=w110) -> (error out=w109:errorcluster)  [unwired: 1 out]
  n164 = Close File(refnum=w116, error in=w109) -> (error out=w41:errorcluster)  [unwired: 1 out]
  n165 = Close File(refnum=w42, error in=w41) -> (error out=w40:errorcluster)  [unwired: 1 out]
  n166 = call-poly <vilib>:"DAQmx Write.vi"("task/channels in"=w78, "data"=0.0, "error in"=w40) -> ("task out"=w77:refnum<k21>, "error out"=w75:errorcluster)  [unwired: 10 in, 1 out]
  n167 = call <vilib>:"DAQmx Stop Task.vi"("task/channels in"=w77, "error in"=w75) -> ("task out"=w76:refnum<k21>, "error out"=w74:errorcluster)  [unwired: 12 in]
  n168 = call <vilib>:"DAQmx Clear Task.vi"("task in"=w76, "error in"=w74) -> ("error out"=w6:errorcluster)  [unwired: 13 in]
  n169 = call <vilib>:"DAQmx Stop Task.vi"("task/channels in"=w58, "error in"=w6) -> ("task out"=w62:refnum<k21>, "error out"=w61:errorcluster)  [unwired: 12 in]
  n170 = call <vilib>:"DAQmx Clear Task.vi"("task in"=w62, "error in"=w61) -> ("error out"=w3:errorcluster)  [unwired: 13 in]
  n171 = call <vilib>:"DAQmx Stop Task.vi"("task/channels in"=w2, "error in"=w3) -> ("task out"=w5:refnum<k21>, "error out"=w4:errorcluster)  [unwired: 12 in]
  n172 = call <vilib>:"DAQmx Clear Task.vi"("task in"=w5, "error in"=w4) -> ("error out"=w1:errorcluster)  [unwired: 13 in]
  n173 = call <vilib>:"Simple Error Handler.vi"("error in (no error)"=w1) -> ()  [unwired: 4 in, 5 out]
